vi "FindModulesInUse.vi"(8 "Error In":errorcluster, 11 "DLL Path":path) -> (0 "Error Out":errorcluster, 1 "Number of Usable Modules":i16 min=0 max=4, 2 "ModuleNoArray":i16[](array[numeric]), 3 "DLL Path":path, 4 "Array Of Serialnumbers":string[](array[string]), 6 "SPCModulesArray":T1[](array[typedef]) {"Bus Number" min=-1 max=255 step=1; "Base I/O Addr" format="%.0x"; "Init Status" min=-10 max=0 step=1; "in Use" min=-1 max=1 step=1; "Slot Number" min=-1 max=255 step=1; "Module Type" items=["SPC-600"=600, "SPC-630"=630, "SPC-700"=700, "SPC-730"=730, "SPC-130"=130, "SPC-830"=830, "SPC-140"=140, "SPC-930"=930, "DPC-230"=230, "SPC-150"=150, "SPC-150 N"=151, "SPC-150 NX"=152, "SPC-130 EM"=131, "SPC-130 EMN"=132, "SPC-160"=160, "SPC-160 X"=161, "SPC-160 PCIE"=162, "SPC-180 N"=180, "SPC-180 NX"=181, "SPC-180 NXX"=182, "SPC-180 N-USB"=185, "SPC-180 NX-USB"=186, "SPC-180 NXX-USB"=187, "TDC-104"=104, "DPC-330"=330, "SPC-590"=590, "Simulation"=-1]})   [LabVIEW 2019]
doc: "This VI is a wrapper for the SPC_get_module_info.vi and SPC_get_eeprom_data.vi and provides the 'SPCModulesArray' and 'Array Of Serialnumbers' for all free SPC modules of possible 32 modules. The amount of currently free modules is counted.\n\ninfo@becker-hickl.com"
uses:
  SPC_Controls/SPCModInfo.ctl
  SPC_Controls/ModuleType.ctl
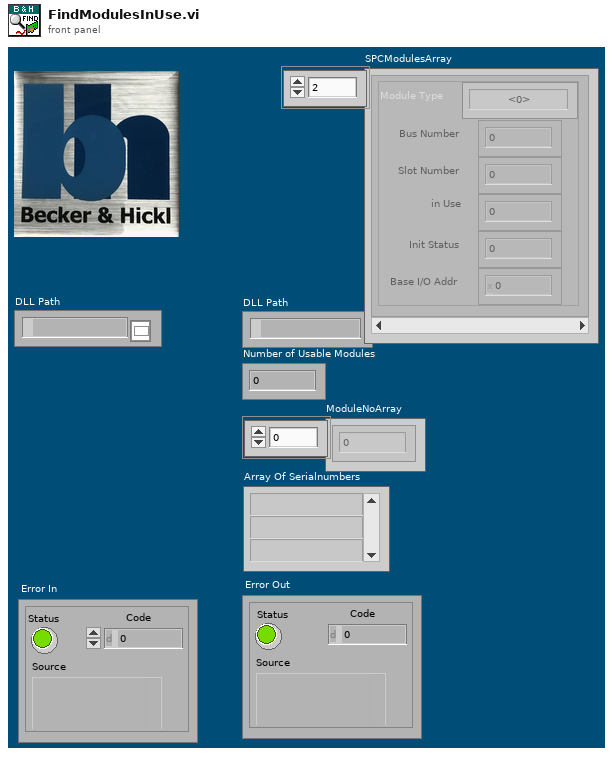
[diagram p1: front panel]
types:
  T1 = typedef "SPCModInfo.ctl" = cluster{"Module Type":T2, "Bus Number":i16, "Slot Number":i16, "in Use":i16, "Init Status":i16, "Base I/O Addr":u16}
  T2 = typedef "ModuleType.ctl" = i16
  T3 = typedef "SPC_eep_data.ctl" = cluster{"module_type[16]":string, "serial_no[16]":string, "date[16]":string, "SPC adjust parameters":T4}
  T4 = typedef "SPC_adjust_para.ctl" = cluster{"vrt1":i16, "vrt2":i16, "vrt3":i16, "dith_g":i16, "gain_1":sgl, "gain_2":sgl, "gain_4":sgl, "gain_8":sgl, "tac_r0":sgl, "tac_r1":sgl, "tac_r2":sgl, "tac_r4":sgl, "tac_r8":sgl, "sync_div":i16}
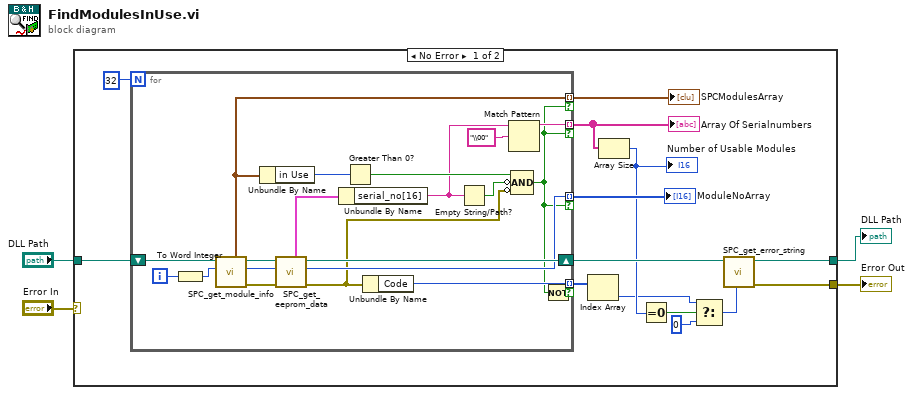
[diagram p0: block diagram]
diagram:
  n1 = case shown="No Error" "Error In" {
    selector: "Error In" -> [_ w40]
    tunnel: "DLL Path" -> [w12 w39]
    tunnel: [w15 w40] -> w3
    tunnel: [w14 w39] -> w2
    frame No Error {
      n2 = for {
        N: 32 ("Element Data") -> [_]
        shift-right: [w30] -> w13
        shift-left: w12 -> [w37]
        tunnel: [w28] -> w7 mode=indexing if=w20
        tunnel: [w27] -> w9 mode=indexing if=w20
        tunnel: [w26] -> w10 mode=indexing if=w20
        tunnel: [w21] -> w6 mode=indexing if=w19
        i -> [w35]
        n3 = To Word Integer(number=w35) -> (16bit integer=w36:i16)
        n4 = call "SPC_get_module_info.vi"("Module No"=w36, "DLL Path"=w37) -> ("Error Out"=w34:errorcluster, "Module No"=w33:i16, "DLL Path"=w32:path, "SPCModInfo"=w26:T1)  [unwired: 6 in]
        n5 = Unbundle By Name(w26) -> ("in Use"=w38:i16)
        n6 = call "SPC_get_eeprom_data.vi"("Error In"=w34, "Module No"=w33, "DLL Path"=w32) -> ("Error Out"=w22:errorcluster, "Module No"=w27:i16, "DLL Path"=w30:path, "SPC EEPROM Data"=w31:T3)  [unwired: 3 in, 2 out]
        n7 = Unbundle By Name(w31) -> ("serial_no[16]"=w23:string)
        n8 = Greater Than 0?(x=w38) -> (x > 0?=w24:bool)
        n9 = Unbundle By Name(w22) -> ("Code"=w21:i32)
        n10 = Empty String/Path?(string/path=w23) -> (empty?=w25:bool)
        n11 = Match Pattern(string=w23, regular expression="\\00") -> (before substring=w28:string)  [unwired: 1 in, 3 out]
        n12 = Compound Arithmetic op=AND(w24, invert w25, invert w22) -> (w20:bool)
        n13 = Not(x=w20) -> (.not. x?=w19:bool)
      }
      "Array Of Serialnumbers" <- w7
      "SPCModulesArray" <- w10
      "ModuleNoArray" <- w9
      n14 = Index Array(array=w6) -> (element=w5:i32)  [unwired: 1 in]
      n15 = Array Size(array=w7) -> (size(s)=w8:i32)
      "Number of Usable Modules" <- w8
      n16 = Equal To 0?(x=w8) -> (x = 0?=w18:bool)
      n17 = Select(t=w5, s=w18, f=i16 0 ("Error code")) -> (s? t:f=w11:i32)
      n18 = call "SPC_get_error_string.vi"("ErrorID"=w11, "DLL Path"=w13) -> ("Error Out"=w15:errorcluster, "DLL Path"=w14:path)  [unwired: 7 in, 1 out]
    }
    frame Error {
    }
  }
  "Error Out" <- w3
  "DLL Path" <- w2
